vi "Horizontal_Move.vi"() -> ()   [LabVIEW 2017]
uses:
  <vilib>/Utility/file.llb/Write Delimited Spreadsheet (DBL).vi
  <vilib>/vision/driver/NI_Vision_Acquisition_Software.lvlib
  <vilib>/vision/NI_Vision_Development_Module.lvlib
panel:
  out "Array":dbl[][](array[numeric])
  out "Boolean 2":bool
  out "X":dbl[](array[numeric])
  out "Numeric 2":dbl
  out "Numeric":dbl
  out "OK Y":dbl
  out "OK X":dbl
  in  "OK Button":bool
  out "Boolean":bool
  out "Y":dbl[](array[numeric])
  out "選擇範圍 2":T1(plugin-control)
  out "error out":errorcluster
  in  "亮度":cluster{"Min":i32, "Max":i32}(slide)={"Min"=60, "Max"=157} scale=0.0..255.0
  in  "飽和度":cluster{"Min":i32, "Max":i32}(slide)={"Min"=0, "Max"=42} scale=0.0..255.0
  in  "色相":cluster{"Min":i32, "Max":i32}(slide)={"Min"=67, "Max"=120} scale=0.0..255.0
  out "顯示錯誤":errorcluster
  out "影像":T1(plugin-control)
  in  "stop":bool
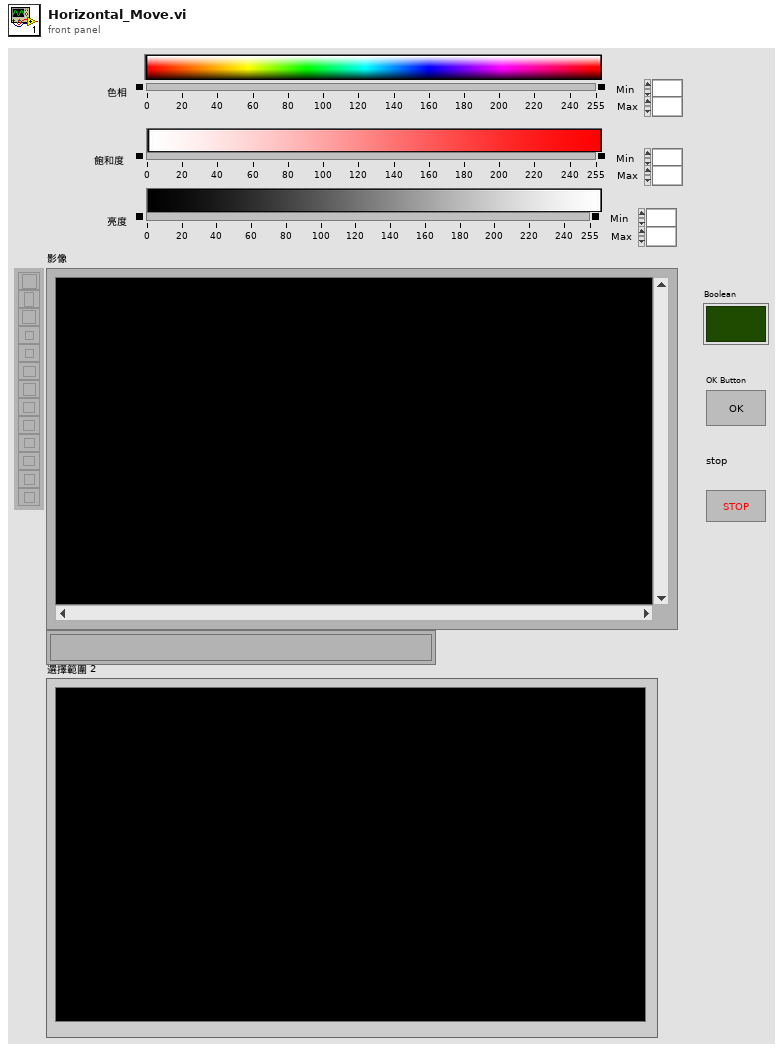
[diagram p1: front panel]
types:
  T1 = typedef "IMAQ Image.ctl" = refnum<image>
  T2 = typedef "Image Type" = u32
  T3 = cluster{"Type":u32, "Version":u32, "Flags":u32, "SerialNumberHigh":u32, "SerialNumberLow":u32, "BusType":u32, "InterfaceName":string, "VendorName":string, "ModelName":string, "CameraFileName":string, "CameraAttributeURL":string}[]
  T4 = cluster{"Type":u32, "Version":u32, "Flags":u32, "SerialNumberHigh":u32, "SerialNumberLow":u32, "BusType":u32, "InterfaceName":string, "VendorName":string, "ModelName":string, "CameraFileName":string, "CameraAttributeURL":string}
  T5 = typedef "IMAQdx.ctl" = refnum<k21>
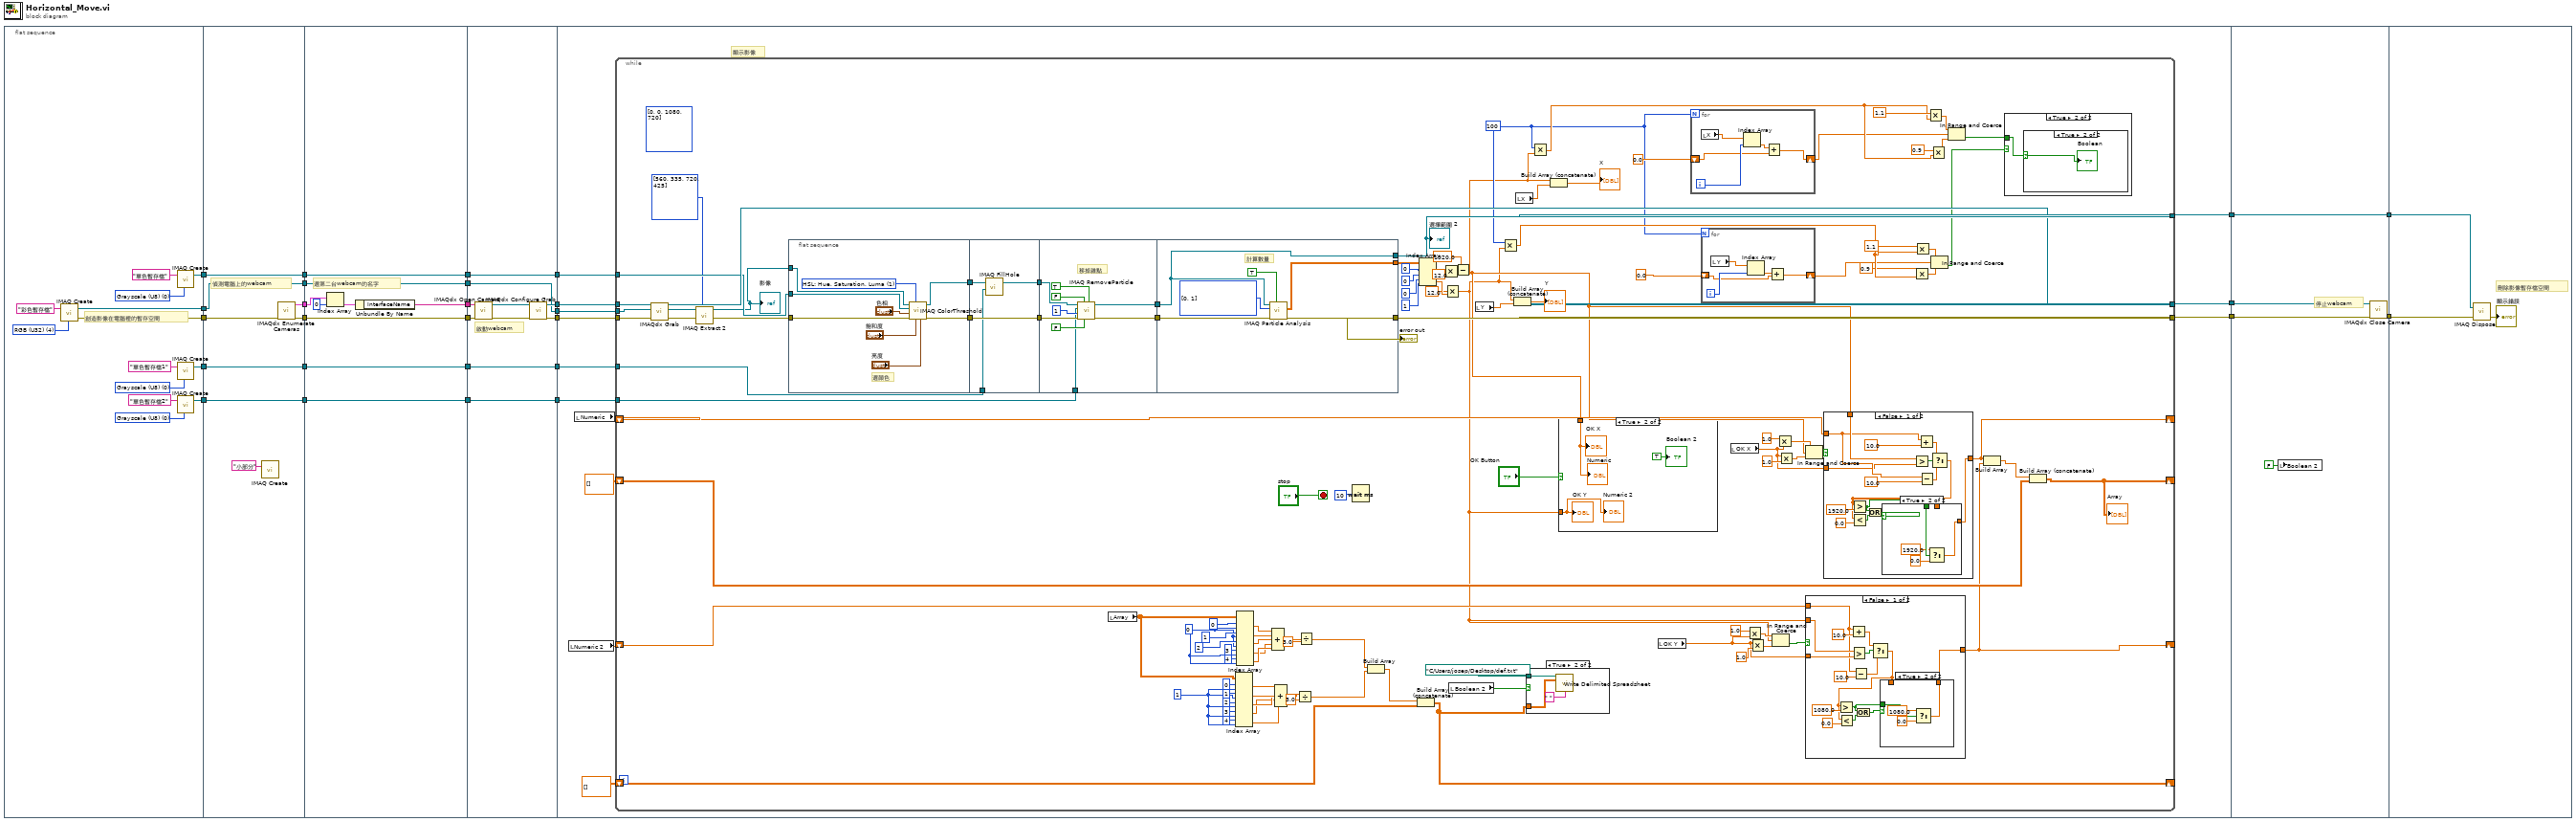
[diagram p0: block diagram]
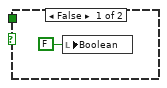
[diagram p3: hidden frame]
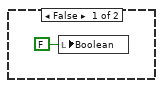
[diagram p4: hidden frame]
diagram:
  n1 = flat-sequence {
    tunnel: [w39] -> w22
    tunnel: [w38] -> w21
    tunnel: [w35] -> w12
    tunnel: [w30] -> w5
    tunnel: [w29] -> w1
    tunnel: [w49] -> w28
    tunnel: [w48] -> w23
    tunnel: w22 -> [w48]
    tunnel: w21 -> [w47]
    tunnel: [w46] -> w19
    tunnel: [w45] -> w13
    tunnel: w12 -> [w45]
    tunnel: [w44] -> w6
    tunnel: w5 -> [w44]
    tunnel: [w43] -> w2
    tunnel: w1 -> [w43]
    tunnel: w28 -> [w56]
    tunnel: [w55] -> w27
    tunnel: [w54] -> w24
    tunnel: w23 -> [w54]
    tunnel: [w53] -> w20
    tunnel: w19 -> [w53]
    tunnel: [w52] -> w14
    tunnel: w13 -> [w52]
    tunnel: [w51] -> w7
    tunnel: w6 -> [w51]
    tunnel: [w50] -> w3
    tunnel: w2 -> [w50]
    tunnel: w27 -> [w67]
    tunnel: [w66] -> w26
    tunnel: [w65] -> w25
    tunnel: w24 -> [w65]
    tunnel: w20 -> [w64]
    tunnel: [w62] -> w18
    tunnel: [w61] -> w15
    tunnel: w14 -> [w61]
    tunnel: [w60] -> w8
    tunnel: w7 -> [w60]
    tunnel: [w59] -> w4
    tunnel: w3 -> [w59]
    tunnel: w26 -> [w81]
    tunnel: w25 -> [w80]
    tunnel: w18 -> [w79]
    tunnel: [w78] -> w16
    tunnel: w15 -> [w77]
    tunnel: [w76] -> w11
    tunnel: [w75] -> w10
    tunnel: w8 -> [w74]
    tunnel: w4 -> [w73]
    tunnel: [w285] -> w17
    tunnel: w16 -> [w284]
    tunnel: w11 -> [w283]
    tunnel: w10 -> [w282]
    tunnel: [w282] -> w9
    tunnel: w17 -> [w288]
    tunnel: w9 -> [w286]
    frame #0 {
      w33 = T2 0 items=["Grayscale (U8)", "Grayscale (I16)", "Grayscale (SGL)", "Complex (CSG)", "RGB (U32)", "HSL (U32)", "RGB (U64)", "Grayscale (U16)"] ("Image Type")
      w34 = T2 0 items=["Grayscale (U8)", "Grayscale (I16)", "Grayscale (SGL)", "Complex (CSG)", "RGB (U32)", "HSL (U32)", "RGB (U64)", "Grayscale (U16)"] ("Image Type")
      w36 = T2 0 items=["Grayscale (U8)", "Grayscale (I16)", "Grayscale (SGL)", "Complex (CSG)", "RGB (U32)", "HSL (U32)", "RGB (U64)", "Grayscale (U16)"] ("Image Type")
      w41 = T2 4 items=["Grayscale (U8)", "Grayscale (I16)", "Grayscale (SGL)", "Complex (CSG)", "RGB (U32)", "HSL (U32)", "RGB (U64)", "Grayscale (U16)"] ("Image Type")
      # "創造影像在電腦裡的暫存空間"
      n2 = call "IMAQ Create"("Image Name"="彩色暫存檔", "Image Type"=w41) -> ("New Image"=w39:T1, "error out"=w38:errorcluster)  [unwired: 3 in]
      n3 = call "IMAQ Create"("Image Name"="單色暫存檔", "Image Type"=w36) -> ("New Image"=w35:T1)  [unwired: 3 in, 1 out]
      n4 = call "IMAQ Create"("Image Name"="單色暫存檔1", "Image Type"=w34) -> ("New Image"=w30:T1)  [unwired: 3 in, 1 out]
      n5 = call "IMAQ Create"("Image Name"="單色暫存檔2", "Image Type"=w33) -> ("New Image"=w29:T1)  [unwired: 3 in, 1 out]
    }
    frame #1 {
      # "偵測電腦上的webcam"
      n6 = call "IMAQ Create"("Image Name"="小部分") -> ()  [unwired: 4 in, 2 out]
      n7 = call <vilib>:"IMAQdx Enumerate Cameras.vi"("error in"=w47) -> ("error out"=w46:errorcluster, "Camera Information Array"=w49:T3)  [unwired: 9 in]
    }
    frame #2 {
      # "選第二台webcam的名字"
      n8 = Index Array(array=w56, index=0) -> (element=w57:T4)
      n9 = Unbundle By Name(w57) -> ("InterfaceName"=w55:string)
    }
    frame #3 {
      # "啟動webcam"
      n10 = call <vilib>:"IMAQdx Open Camera.vi"("error in"=w64, "Session In"=w67) -> ("error out"=w63:errorcluster, "Session Out"=w68:T5)  [unwired: 8 in]
      n11 = call <vilib>:"IMAQdx Configure Grab.vi"("error in"=w63, "Session In"=w68) -> ("error out"=w62:errorcluster, "Session Out"=w66:T5)  [unwired: 8 in]
    }
    frame #4 {
      # "顯示影像"
      n12 = local read "Numeric 2"() -> (w71:dbl)
      n13 = local read "Numeric"() -> (w72:dbl)
      n14 = while {
        tunnel: w81 -> [w189]
        tunnel: w80 -> [w126]
        tunnel: w79 -> [w188]
        tunnel: [w187] -> w78
        tunnel: w77 -> [w176]
        tunnel: [w178] -> w76
        tunnel: [w177] -> w75
        tunnel: w74 -> [w171]
        tunnel: w73 -> [w170]
        shift-right: [w127] -> _
        shift-left: w72 -> [w152]
        shift-right: [w128] -> _
        shift-left: w71 -> [w142]
        shift-right: [w115] -> _
        shift-left: dbl[][] [] -> [w143]
        shift-right: [w101] -> _
        shift-left: dbl[][] [] -> [w102]
        stop <- "stop" stop-if-true
        w91 = 1 ("disabled index (col)")
        w90 = 0 ("disabled index (col)")
        (unwired) i32[] [0, 0, 1080, 720] ("Optional Rectangle")
        w123 = 100
        n15 = call <vilib>:"IMAQdx Grab.vi"("error in"=w188, "Image In"=w126, "Session In"=w189) -> ("error out"=w180:errorcluster, "Image Out"=w125:T1, "Session Out"=w187:T5)  [unwired: 5 in, 1 out]
        n16 = call "IMAQ Extract 2"("Optional Rectangle"=i32[] [560, 335, 720, 425], "Image Src"=w125) -> ("Image Dst Out"=w124:T1)  [unwired: 8 in, 1 out]
        "影像" <- w124
        n17 = flat-sequence {
          tunnel: w180 -> [w255]
          tunnel: w124 -> [w257]
          tunnel: [w254] -> w174
          tunnel: w176 -> [w256]
          tunnel: [w253] -> w172
          tunnel: [w263] -> w175
          tunnel: w174 -> [w265]
          tunnel: [w265] -> w173
          tunnel: w172 -> [w264]
          tunnel: w171 -> [w262]
          tunnel: [w268] -> w182
          tunnel: [w267] -> w181
          tunnel: w175 -> [w270]
          tunnel: w173 -> [w269]
          tunnel: w170 -> [w266]
          tunnel: [w279] -> w177
          tunnel: [w275] -> w178
          tunnel: w182 -> [w278]
          tunnel: w181 -> [w279]
          tunnel: [w276] -> w179
          frame #0 {
            w258 = 1 items=["RGB (Red, Green, Blue)", "HSL: Hue, Saturation, Luma"] ("Threshold Color Mode")
            # "選顏色"
            n18 = call "IMAQ ColorThreshold"("Blue or Luma or Val or Inten Range"="亮度", "Green or Sat Range"="飽和度", "Color Mode"=w258, "error in (no error)"=w255, "Red or Hue Range"="色相", "Image Dst"=w256, "Image Src"=w257) -> ("error out"=w254:errorcluster, "Image Dst Out"=w253:T1)  [unwired: 1 in, 2 out]
          }
          frame #1 {
            n19 = call "IMAQ FillHole"("Image Dst"=w262, "Image Src"=w264) -> ("Image Dst Out"=w263:T1)  [unwired: 2 in, 3 out]
          }
          frame #2 {
            # "移掉雜點"
            n20 = call "IMAQ RemoveParticle"("Connectivity 4/8 (8)"=TRUE, "Low Pass/High Pass (Low)"=FALSE, "Square/Hexa (Square)"=FALSE, "error in (no error)"=w269, "Number of Erosion"=1, "Image Dst"=w266, "Image Src"=w270) -> ("error out"=w268:errorcluster, "Image Dst Out"=w267:T1)  [unwired: 3 out]
          }
          frame #3 {
            w277 = i32[] [0, 1] items=["Center of Mass X", "Center of Mass Y", "First Pixel X", "First Pixel Y", "Bounding Rect Left", "Bounding Rect Top", "Bounding Rect Right", "Bounding Rect Bottom", "Max Feret Diameter Start X", "Max Feret Diameter Start Y", "Max Feret Diameter End X", "Max Feret Diameter End Y", "Max Horiz. Segment Length Left", "Max Horiz. Segment Length Right", "Max Horiz. Segment Length Row", "-", "Bounding Rect Width", "Bounding Rect Height", "Bounding Rect Diagonal", "Perimeter", "Convex Hull Perimeter", "Holes' Perimeter", "Max Feret Diameter", "Equivalent Ellipse Major Axis", "Equivalent Ellipse Minor Axis", "Equivalent Ellipse Minor Axis (Feret)", "Equivalent Rect Long Side", "Equivalent Rect Short Side", "Equivalent Rect Diagonal", "Equivalent Rect Short Side (Feret)", "Average Horiz. Segment Length", "Average Vert. Segment Length", "Hydraulic Radius", "Waddel Disk Diameter", "-", "Area", "Holes' Area", "Particle & Holes' Area", "Convex Hull Area", "Image Area", "-", "Number of Holes", "Number of Horiz. Segments", "Number of Vert. Segments", "-", "Orientation", "Max Feret Diameter Orientation", "-", "% Area/Image Area", "% Area/(Particle & Holes' Area)", "Ratio of Equivalent Ellipse Axes", "Ratio of Equivalent Rect Sides", "-", "Elongation Factor", "Compactness Factor", "Heywood Circularity Factor", "Type Factor", "-", "Sum X", "Sum Y", "Sum XX", "Sum XY", "Sum YY", "Sum XXX", "Sum XXY", "Sum XYY", "Sum YYY", "-", "Moment of Inertia XX", "Moment of Inertia XY", "Moment of Inertia YY", "Moment of Inertia XXX", "Moment of Inertia XXY", "Moment of Inertia XYY", "Moment of Inertia YYY", "Norm. Moment of Inertia XX", "Norm. Moment of Inertia XY", "Norm. Moment of Inertia YY", "Norm. Moment of Inertia XXX", "Norm. Moment of Inertia XXY", "Norm. Moment of Inertia XYY", "Norm. Moment of Inertia YYY", "Hu Moment 1", "Hu Moment 2", "Hu Moment 3", "Hu Moment 4", "Hu Moment 5", "Hu Moment 6", "Hu Moment 7"] ("Pixel Measurements")
            # "計算數量"
            n21 = call "IMAQ Particle Analysis"("Connectivity 4/8 (8)"=TRUE, "error in (no error)"=w278, "Pixel Measurements"=w277, "Image"=w279) -> ("error out"=w275:errorcluster, "Particle Measurements (Pixels)"=w276:dbl[][])  [unwired: 1 in, 5 out]
          }
        }
        n22 = local read "Array"() -> (w114:dbl[][])
        n23 = Index Array(array=w114, index (row) #1=0 ("disabled index (row)"), index (col) #1=w91, index (row) #2=1 ("disabled index (row)"), index (col) #2=w91, index (row) #3=2 ("disabled index (row)"), index (col) #3=w91, index (row) #4=3 ("disabled index (row)"), index (col) #4=w91, index (row) #5=4 ("disabled index (row)"), index (col) #5=w91) -> (element #1=w110:dbl, element #2=w109:dbl, element #3=w108:dbl, element #4=w83:dbl, element #5=w82:dbl)
        n24 = Index Array(array=w114, index (row) #1=0 ("disabled index (row)"), index (col) #1=w90, index (row) #2=1 ("disabled index (row)"), index (col) #2=w90, index (row) #3=2 ("disabled index (row)"), index (col) #3=w90, index (row) #4=3 ("disabled index (row)"), index (col) #4=w90, index (row) #5=4 ("disabled index (row)"), index (col) #5=w90) -> (element #1=w113:dbl, element #2=w112:dbl, element #3=w111:dbl, element #4=w84:dbl, element #5=w85:dbl)
        n25 = Compound Arithmetic op=ADD(w113, w112, w111, w84, w85) -> (w106:dbl)
        n26 = Compound Arithmetic op=ADD(w110, w109, w108, w83, w82) -> (w105:dbl)
        n27 = Divide(x=w105, y=3.0) -> (x/y=w98:dbl)
        n28 = Divide(x=w106, y=3.0) -> (x/y=w99:dbl)
        n29 = Wait (ms)(milliseconds to wait=u32 10 ("millisecond timer value")) -> ()  [unwired: 1 out]
        n30 = Build Array(w99, w98) -> (w103:dbl[])
        n31 = Build Array (concatenate)(w103, w102) -> (w101:dbl[][])
        n32 = Index Array(array=w179, index (row) #1=0 ("disabled index (row)"), index (col) #1=0 ("disabled index (col)"), index (row) #2=0 ("index (row)"), index (col) #2=1 ("disabled index (col)")) -> (element #1=w138:dbl, element #2=w141:dbl)
        n33 = Multiply(x=w138, y=12.0) -> (x*y=w122:dbl)
        n34 = Multiply(x=12.0, y=w141) -> (x*y=w116:dbl)
        n35 = local read "Boolean 2"() -> (w119:bool)
        n36 = Subtract(x=1920.0, y=w122) -> (x-y=w118:dbl)
        n37 = local read "Y"() -> (w168:dbl[])
        n38 = Multiply(x=w123, y=w116) -> (x*y=w163:dbl)
        n39 = Build Array (concatenate)(w116, w168) -> (→"Y":dbl[])
        n40 = local read "X"() -> (w139:dbl[])
        n41 = case shown="True" w119 {
          tunnel: path "C:/Users/josep/Desktop/def.txt" ("file path (dialog if empty)") -> [_ w193]
          tunnel: w101 -> [_ w191]
          frame False {
          }
          frame True {
            n42 = call-poly <vilib>:"Write Delimited Spreadsheet.vi"("file path (dialog if empty)"=w193, "2D data"=w191, "delimiter (\\t)"=" " ("delimiter (\\t)")) -> ()  [unwired: 11 in, 2 out]
          }
        }
        n43 = Multiply(x=w123, y=w118) -> (x*y=w132:dbl)
        n44 = Build Array (concatenate)(w118, w139) -> (→"X":dbl[])
        n45 = case shown="True" "OK Button" {
          tunnel: w118 -> [_ w246]
          tunnel: w116 -> [_ w247]
          frame False {
          }
          frame True {
            "OK X" <- w246
            "OK Y" <- w247
            "Numeric" <- w246
            "Numeric 2" <- w247
            "Boolean 2" <- TRUE ("Boolean 2")
          }
        }
        n46 = local read "OK Y"() -> (w145:dbl)
        n47 = for {
          N: w123 -> [_]
          shift-right: [w199] -> w131
          shift-left: 0.0 -> [w198]
          i -> [w201]
          n48 = local read "X"() -> (w202:dbl[])
          n49 = Index Array(array=w202, index=w201) -> (element=w200:dbl)
          n50 = Add(x=w200, y=w198) -> (x+y=w199:dbl)
        }
        n51 = for {
          N: w123 -> [_]
          shift-right: [w249] -> w162
          shift-left: 0.0 -> [w248]
          i -> [w251]
          n52 = local read "Y"() -> (w252:dbl[])
          n53 = Index Array(array=w252, index=w251) -> (element=w250:dbl)
          n54 = Add(x=w250, y=w248) -> (x+y=w249:dbl)
        }
        n55 = local read "OK X"() -> (w151:dbl)
        n56 = Multiply(x=1.0, y=w145) -> (x*y=w149:dbl)
        n57 = Multiply(x=w145, y=1.0) -> (x*y=w148:dbl)
        n58 = In Range and Coerce(upper limit=w149, x=w116, lower limit=w148) -> (In Range?=w150:bool)  [unwired: 1 out]
        n59 = Multiply(x=1.0, y=w151) -> (x*y=w154:dbl)
        n60 = Multiply(x=w151, y=1.0) -> (x*y=w153:dbl)
        n61 = In Range and Coerce(upper limit=w154, x=w118, lower limit=w153) -> (In Range?=w157:bool)  [unwired: 1 out]
        n62 = case shown="False" w150 {
          tunnel: [w204 w223] -> w128
          tunnel: w145 -> [w212 _]
          tunnel: w116 -> [w211 w223]
          tunnel: w142 -> [w210 _]
          frame False {
            n63 = Add(x=w210, y=10.0) -> (x+y=w217:dbl)
            n64 = Greater?(x=w211, y=w212) -> (0:w213:bool)
            n65 = Subtract(x=w210, y=10.0) -> (x-y=w216:dbl)
            n66 = Select(t=w217, s=w213, f=w216) -> (s? t:f=w203:dbl)
            n67 = Greater?(x=w203, y=1080.0) -> (0:w205:bool)
            n68 = Less?(x=w203, y=0.0) -> (x < y?=w208:bool)
            n69 = Or(x=w205, y=w208) -> (x .or. y?=w209:bool)
            n70 = case shown="True" w209 {
              tunnel: w205 -> [_ w222]
              tunnel: w203 -> [w218 _]
              tunnel: [w218 w219] -> w204
              frame False {
              }
              frame True {
                n71 = Select(t=1080.0, s=w222, f=0.0) -> (s? t:f=w219:dbl)
              }
            }
          }
          frame True {
          }
        }
        n72 = case shown="False" w157 {
          tunnel: [w226 w244] -> w127
          tunnel: w118 -> [w237 _]
          tunnel: w152 -> [w232 w244]
          tunnel: w151 -> [w231 _]
          frame False {
            n73 = Greater?(x=w237, y=w231) -> (0:w238:bool)
            n74 = Add(x=w232, y=10.0) -> (x+y=w233:dbl)
            n75 = Subtract(x=w232, y=10.0) -> (x-y=w234:dbl)
            n76 = Select(t=w233, s=w238, f=w234) -> (s? t:f=w224:dbl)
            n77 = Greater?(x=w224, y=1920.0) -> (0:w225:bool)
            n78 = Less?(x=w224, y=0.0) -> (x < y?=w230:bool)
            n79 = Or(x=w225, y=w230) -> (x .or. y?=w227:bool)
            n80 = case shown="True" w227 {
              tunnel: [w239 w240] -> w226
              tunnel: w224 -> [w239 _]
              tunnel: w225 -> [_ w243]
              frame False {
              }
              frame True {
                n81 = Select(t=1920.0, s=w243, f=0.0) -> (s? t:f=w240:dbl)
              }
            }
          }
          frame True {
          }
        }
        n82 = Multiply(x=0.9, y=w163) -> (x*y=w164:dbl)
        n83 = Multiply(x=1.1, y=w163) -> (x*y=w165:dbl)
        n84 = Multiply(x=1.1, y=w132) -> (x*y=w136:dbl)
        n85 = Multiply(x=0.9, y=w132) -> (x*y=w135:dbl)
        n86 = In Range and Coerce(upper limit=w165, x=w162, lower limit=w164) -> (In Range?=w130:bool)  [unwired: 1 out]
        n87 = In Range and Coerce(upper limit=w136, x=w131, lower limit=w135) -> (In Range?=w129:bool)  [unwired: 1 out]
        n88 = Build Array(w127, w128) -> (w144:dbl[])
        n89 = case shown="True" w130 {
          tunnel: w129 -> [_ w195]
          frame False {
            n90 = local write "Boolean"(FALSE ("Boolean")) -> ()
          }
          frame True {
            n91 = case shown="True" w195 {
              selector: w195 -> [_ w197]
              frame False {
                n92 = local write "Boolean"(FALSE ("Boolean")) -> ()
              }
              frame True {
                "Boolean" <- w197
              }
            }
          }
        }
        n93 = Build Array (concatenate)(w144, w143) -> (w115:dbl[][])
        "Array" <- w115
        "error out" <- w178
        "選擇範圍 2" <- w177
      }
    }
    frame #5 {
      # "停止webcam"
      n94 = local write "Boolean 2"(FALSE ("Boolean 2")) -> ()
      n95 = call <vilib>:"IMAQdx Close Camera.vi"("error in"=w283, "Session In"=w284) -> ("error out"=w285:errorcluster)  [unwired: 9 in]
    }
    frame #6 {
      # "刪除影像暫存檔空間"
      n96 = call "IMAQ Dispose"("Image"=w286, "error in (no error)"=w288) -> ("error out"=→"顯示錯誤":errorcluster)  [unwired: 4 in]
    }
  }
